vi "SPA_Hex_String.vi"(0 "System no.":i32=1 min=1 max=4 step=1, 2 "Designator to set":string[](array[string]), 3 "Parameter string":string[](array[string]), 5 "error in":errorcluster, 6 "Parameter number (hex)":u32[](array[numeric]) format="%.0x") -> (14 "Controller error":bool, 19 "error out":errorcluster)   [LabVIEW 2026]
doc: "Sets string parameters for commanded designators, waits 100 ms and queries ERR?. For axis-related parameters, Designator to set is the axis name; for piezo- or sensor-related parameters, the channel number, otherwise a parameter-related one. Controller error is TRUE if selected system reports an error code which is not 0. For parameter numbers which require a numerical value as input use SPA_hex.vi. See GCS DLL manual for available parameter numbers.\nOld VI - please use SPA.vi instead."
panel:
  # "This vi sets string parameters for commanded designators, waits 100 ms and queries ERR?. \nSee GCS DLL manual for available parameter numbers and strings. For parameter numbers \nwhich require a numerical value as input use \"SPA_hex.vi\".\nOld VI - please use SPA.vi instead."
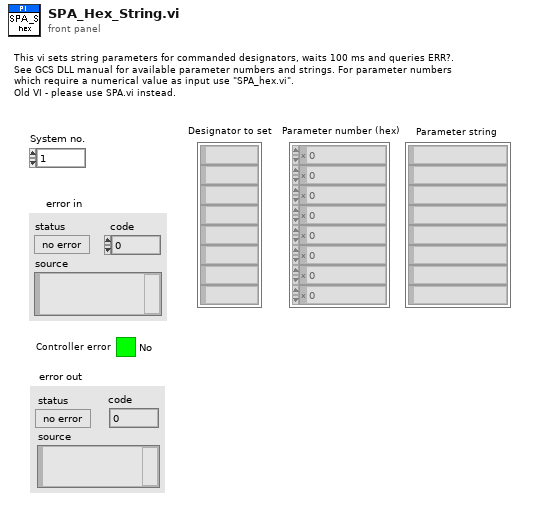
[diagram p1: front panel]
types:
  T1 = enum16{"Disable error check", "Force error check", "Use global settings"}
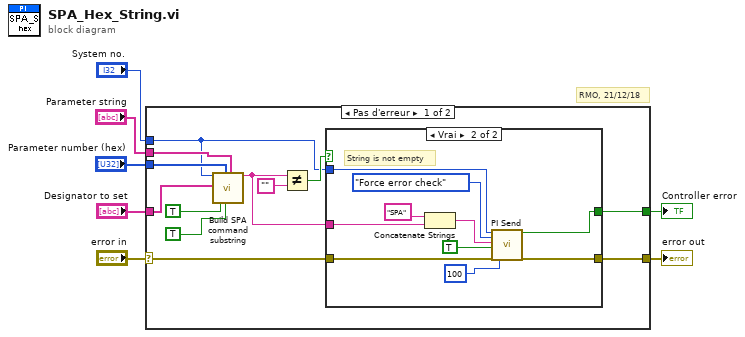
[diagram p0: block diagram]
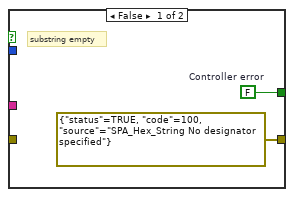
[diagram p2: hidden frame]
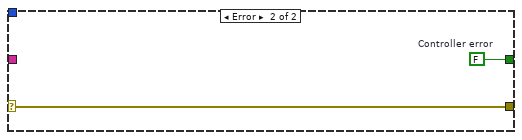
[diagram p3: hidden frame]
diagram:
  # "RMO, 21/12/18"
  n1 = case shown="Pas d'erreur" "error in" {
    selector: "error in" -> [w9 w33]
    tunnel: [w19 w33] -> w7
    tunnel: "Parameter string" -> [w13 _]
    tunnel: "System no." -> [w12 _]
    tunnel: "Designator to set" -> [w16 _]
    tunnel: "Parameter number (hex)" -> [w15 _]
    tunnel: [w8 w32] -> w1
    frame No Error {
      n2 = call "Build SPA command substring.vi"("System no."=w12, "Axes to set"=w16, "Parameter no. format \n(Decimal: FALSE)"=TRUE ("Parameter no. format \n(Decimal: FALSE)"), "Parameter number (hex)"=w15, "Parameter format \n(Num.: FALSE)"=TRUE ("Parameter format \n(Num.: FALSE)"), "Parameter strings"=w13) -> ("SPA command substring"=w17:string)  [unwired: 4 in, 9 out]
      n3 = Not Equal?(x=w17, y="") -> (x != y?=w14:bool)
      n4 = case shown="Vrai" w14 {
        tunnel: w17 -> [_ w30]
        tunnel: [errorcluster {"status"=TRUE, "code"=100, "source"="SPA_Hex_String No designator specified"} ("error out") w24] -> w19
        tunnel: w9 -> [_ w27]
        tunnel: w12 -> [_ w26]
        tunnel: [w20 w22] -> w8
        frame False {
          w20 = FALSE  # Controller error
          # "substring empty"
        }
        frame True {
          # "String is not empty"
          n5 = Concatenate Strings("SPA", w30) -> (w28:string)
          n6 = call "PI Send.vi"("System no."=w26, "Error check settings"=T1."Force error check", "String to send"=w28, "Attach termination char.?"=TRUE ("Attach Linefeed?"), "error in"=w27, "Delay before error check (ms)"=u32 100 ("milliseconds to wait")) -> ("Controller error"=w22:bool, "error out"=w24:errorcluster)  [unwired: 12 out]
        }
      }
    }
    frame Error {
      w32 = FALSE  # Controller error
    }
  }
  "error out" <- w7
  "Controller error" <- w1
